vi "Make lots of wires.vi"(8 "error in":errorcluster, 10 "Wire Temrinals 2":refnum<vi>[](array[refnum]), 11 "Wire Terminals 1":refnum<vi>[](array[refnum])) -> (0 "error out":errorcluster, 3 "Wire Sink Terminals":refnum<vi>[](array[refnum]))   [LabVIEW 2012, in "Scripting Tools.lvlib"]
doc: "Make a set of wires between <b>Wire Terminals 1</b> and <bWire Terminals 2</b>, returning references to the sink terminals of the wires."
uses:
  Scripting Tools.lvlib
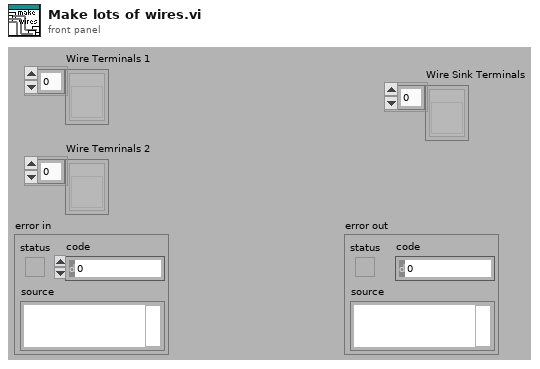
[diagram p1: front panel]
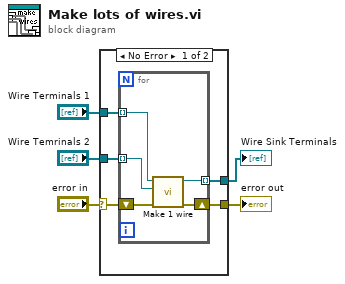
[diagram p0: block diagram]
diagram:
  n1 = case shown="No Error" "error in" {
    selector: "error in" -> [w9 w16]
    tunnel: [w10 w16] -> w5
    tunnel: [w8 _] -> w3
    tunnel: "Wire Temrinals 2" -> [w7 _]
    tunnel: "Wire Terminals 1" -> [w6 _]
    frame No Error {
      n2 = for {
        shift-right: [w14] -> w10
        shift-left: w9 -> [w15]
        tunnel: [w11] -> w8 mode=indexing
        tunnel: w7 -> [w13] mode=indexing
        tunnel: w6 -> [w12] mode=indexing
        n3 = call "Make 1 wire.vi"("error in"=w15, "Wire Terminal 2"=w13, "Wire Terminal 1"=w12) -> ("error out"=w14:errorcluster, "Wire Sink Terminal Out"=w11:refnum<vi>)  [unwired: 7 out]
      }
    }
    frame Error {
    }
  }
  "error out" <- w5
  "Wire Sink Terminals" <- w3
